vi "Test Matrix Solution.vi"() -> ()   [LabVIEW 2013]
uses:
  <vilib>/Analysis/7linalg.llb/Solve Linear Equations (single right hand).vi
  <vilib>/Analysis/baseanly.llb/Solve Linear Equations By Cholesky.vi
  <vilib>/Analysis/baseanly.llb/Real Matrix to Compact Array.vi
  <vilib>/Analysis/baseanly.llb/Real Compact Tri-Matrix Linear Eqs.vi
  <vilib>/Analysis/Matrix/Numeric/Conversions/Array To Matrix - RA2.vi
  <vilib>/Analysis/7linalg.llb/Solve Linear Eqs (General).vi
  <vilib>/Analysis/7linalg.llb/Solve Linear Eqs (Gen, single right hand).vi
  <vilib>/Analysis/NI_AALPro.lvlib
  <vilib>/Analysis/Matrix/NI_Matrix.lvlib
panel:
  out "Solution Vector":dbl[](array[numeric]) format="%.2f"
  out "direct solution":dbl[](array[numeric]) format="%.2f"
  in  "x":i64[](array[numeric])=[0, 0, 0]
  out "inv(A)":dbl[](array[numeric])
  out "cof(A)T":i64[](array[numeric])
  out "cofA":i64[](array[numeric])
  out "det(A)":i64
  in  "A":i64[](array[numeric])=[0, 0, 0, 0, 0, 0, 0, 0, 0]
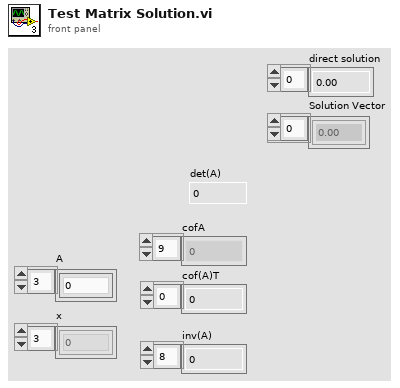
[diagram p1: front panel]
types:
  T1 = typedef "NI_Matrix.lvlib/RealMatrix.ctl" = dbl[][]
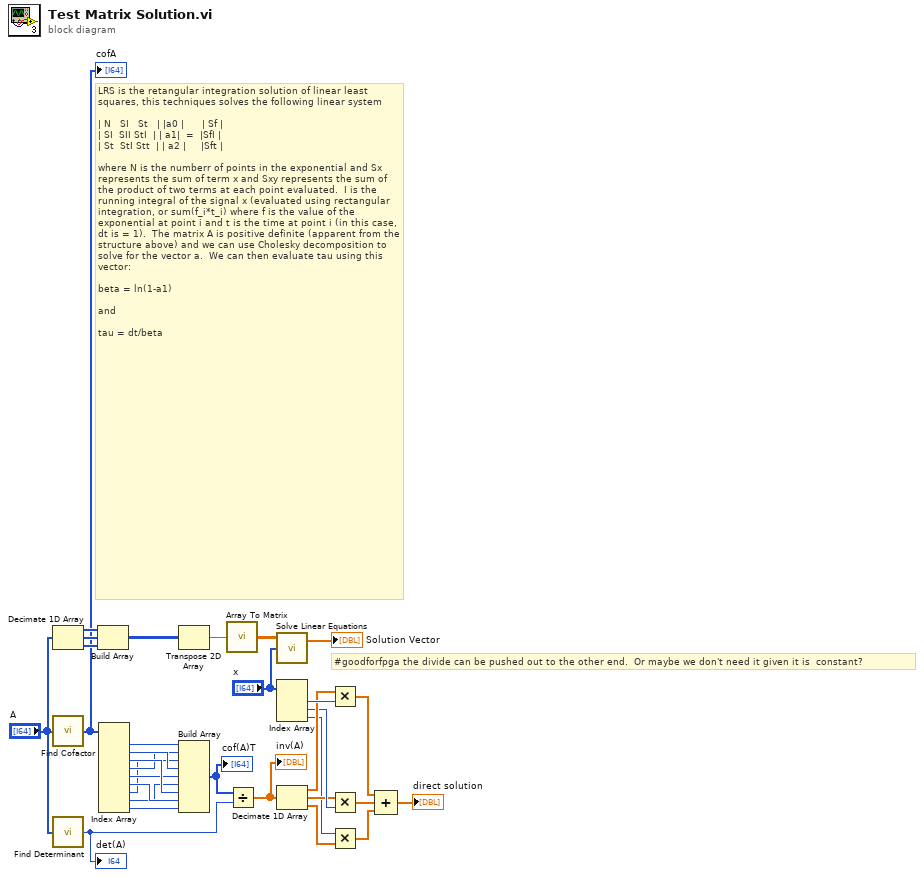
[diagram p0: block diagram]
diagram:
  # "#goodforfpga the divide can be pushed out to the other end.  Or maybe we don't need it given it is  constant?"
  # "LRS is the retangular integration solution of linear least squares, this techniques solves the following linear system \n\n| N   SI   St   | |a0 |      | Sf |\n| SI  SII StI  | | a1|  =  |SfI |\n| St  StI Stt  | | a2 |     |Sft |\n\nwhere N is the numberr of points in the exponential and Sx represents the sum of term x and Sxy represents the sum of the product of two terms at each point evaluated.  I is the running integral of the signal x (evaluated using rectangular integration, or sum(f_i*t_i) where f is the value of the exponential at point i and t is the time at point i (in this case, dt is = 1).  The matrix A is positive definite (apparent from the structure above) and we can use Cholesky decomposition to solve for the vector a.  We can then evaluate tau using this vector:\n\nbeta = ln(1-a1)\n\nand \n\ntau = dt/beta"
  n1 = Decimate 1D Array("A") -> (w9:i64[], w8:i64[], w7:i64[])
  n2 = call "Find Cofactor.vi"("A"="A") -> ("cofA"=w5:i64[])  [unwired: 4 in]
  "cofA" <- w5
  n3 = call "Find Determinant.vi"("A"="A") -> ("det(A)"=w2:i64)  [unwired: 4 in]
  "det(A)" <- w2
  n4 = Build Array(w9, w8, w7) -> (w21:i64[][])
  n5 = Index Array(array=w5) -> (element #1=w18:i64, element #2=w17:i64, element #3=w16:i64, element #4=w15:i64, element #5=w14:i64, element #6=w13:i64, element #7=w12:i64, element #8=w11:i64, element #9=w10:i64)  [unwired: 9 in]
  n6 = Transpose 2D Array(2D array=w21) -> (transposed array=w20:i64[][])
  n7 = Build Array(w18, w15, w12, w17, w14, w11, w16, w13, w10) -> (w4:i64[])
  "cof(A)T" <- w4
  n8 = call-poly <vilib>:"Array To Matrix.vi"("Real 2D Array"=w20) -> ("Real Matrix"=w23:T1)
  n9 = Divide(x=w4, y=w2) -> (x/y=w1:dbl[])
  "inv(A)" <- w1
  n10 = call-poly <vilib>:"Solve Linear Equations.vi"("Known Vector"="x", "Input Matrix"=w23) -> ("Solution Vector"=→"Solution Vector":dbl[])  [unwired: 1 in, 1 out]
  n11 = Index Array(array="x") -> (element #1=w32:i64, element #2=w30:i64, element #3=w27:i64)  [unwired: 3 in]
  n12 = Decimate 1D Array(w1) -> (w31:dbl[], w29:dbl[], w28:dbl[])
  n13 = Multiply(x=w31, y=w32) -> (x*y=w26:dbl[])
  n14 = Multiply(x=w29, y=w30) -> (x*y=w25:dbl[])
  n15 = Multiply(x=w27, y=w28) -> (x*y=w24:dbl[])
  n16 = Compound Arithmetic op=ADD(w26, w25, w24) -> (→"direct solution":dbl[])
